vi "Teleop - Save Maximum Value (SubVI).vi"(10 "Velocity (Raw Sensor Units per 100 ms) in":i32, 11 "Reset Value":bool) -> (3 "Velocity (Raw Sensor Units per 100 ms) out":i32)   [LabVIEW 2019]
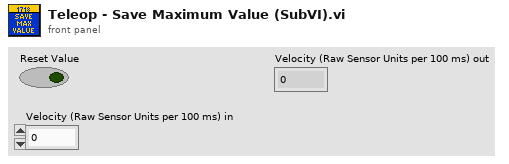
[diagram p1: front panel]
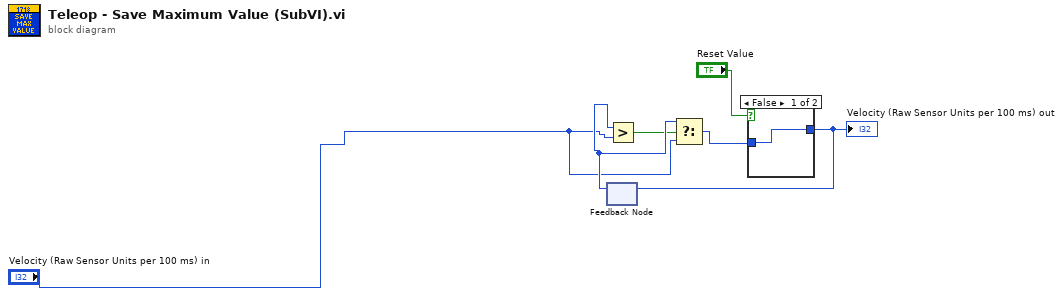
[diagram p0: block diagram]
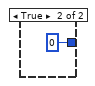
[diagram p2: hidden frame]
diagram:
  n1 = feedback #1() -> (w6:i32)  [unwired: 1 in]
  n2 = Greater?(x=w6, y="Velocity (Raw Sensor Units per 100 ms) in") -> (0:w1:bool)
  n3 = Select(t=w6, s=w1, f="Velocity (Raw Sensor Units per 100 ms) in") -> (s? t:f=w4:i32)
  n4 = case shown="False" "Reset Value" {
    tunnel: w4 -> [w7 _]
    tunnel: [w7 0 ("Velocity (Raw Sensor Units per 100 ms)")] -> w3
    frame False {
    }
    frame True {
    }
  }
  "Velocity (Raw Sensor Units per 100 ms) out" <- w3
  n5 = feedback-in #1(w3) -> ()
